vi "DAQ_Control.vi"(0 "Channel in":T3, 3 "Reading Cluster in":T1, 4 "Iteration Duration":i64) -> (5 "DAQ time":u32, 6 "Gradients":waveform(dbl)[](graph), 7 "cDAQ time":u32, 9 "Stop?":bool, 10 "Temps":waveform(dbl)[](graph), 11 "Time Left:":string, 12 "Camera Feed":T5, 13 "Output%":dbl(slide) caption="Cooling" scale=0.0..100.0 scale format="%.0f %", 14 "Channel out":T4, 15 "Readings out":T2, 17 "Reading Cluster":T1, 18 "DP_Overhead":i64(graph) caption="Data Acquisition - Overhead", 19 "Temp":dbl[unit] caption="Temperature" format="%.2f")   [LabVIEW 2024]
uses:
  <vilib>/vision/Image Controls.llb/IMAQ Image.ctl
  <extravilib>/ChannelInstances/Stream-str/)Channel.ctl
  <extravilib>/ChannelInstances/Tag-t'DataCluster.ctl'/))Channel.ctl
  DataCluster.ctl
  <vilib>/userDefined/High Color/IMAQdx.ctl
  <extravilib>/ChannelInstances/Tag-c(a[.](dbl),a[.](dbl))/))Channel.ctl
  <extravilib>/ChannelInstances/Tag-t'DataCluster.ctl'/Read With Abort.vi
  <extravilib>/ChannelInstances/Tag-c(a[.](dbl),a[.](dbl))/Write With Abort.vi
  <extravilib>/ChannelInstances/Tag-t'DataCluster.ctl'/EndpointRead.vi
  <extravilib>/ChannelInstances/Tag-c(a[.](dbl),a[.](dbl))/Endpoint.vi
  <extravilib>/ChannelInstances/Tag-t'DataCluster.ctl'.lvlib
  <extravilib>/ChannelInstances/Tag-c(a[.](dbl),a[.](dbl)).lvlib
  <extravilib>/ChannelInstances/Stream-str.lvlib
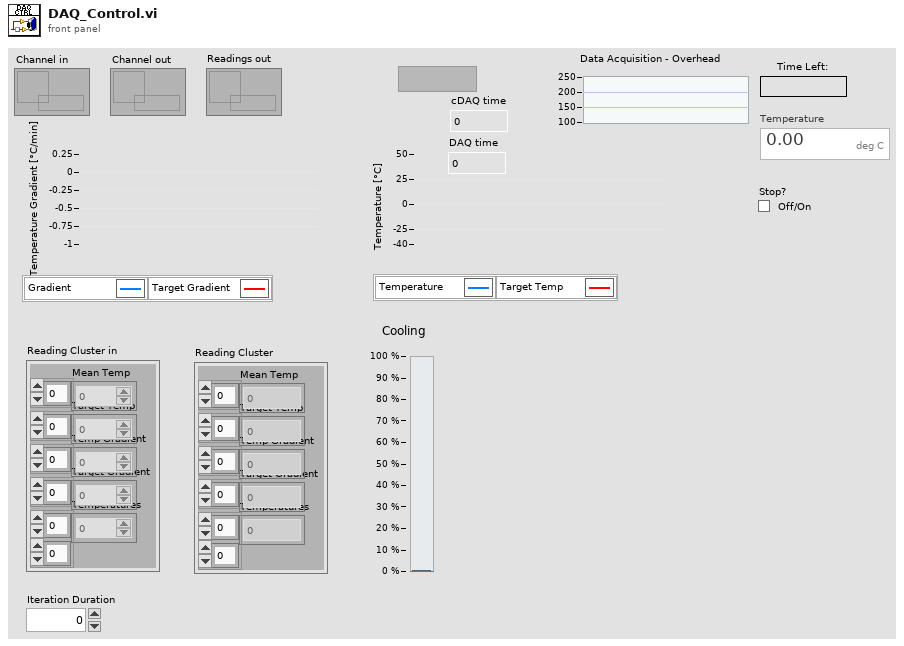
[diagram p1: front panel]
types:
  T1 = cluster{"Mean Temp":dbl[], "Target Temp":dbl[], "Temp Gradient":dbl[], "Target Gradient":dbl[], "Temperatures":dbl[][]}
  T2 = typedef "Tag-c(a[.](dbl),a[.](dbl)).lvlib/))Channel.ctl" = refnum<queue>
  T3 = typedef "Tag-t'DataCluster.ctl'.lvlib/))Channel.ctl" = refnum<queue>
  T4 = typedef "Stream-str.lvlib/)Channel.ctl" = refnum<queue>
  T5 = typedef "IMAQ Image.ctl" = refnum<image>
  T6 = typedef "DataCluster.ctl" = cluster{"Core":cluster{"Current VI Reference":refnum<vi>, "Close Panel on Exit?":bool, "Exit":bool, "Initialized?":bool}, "Connections":cluster{"cDAQ":cluster{"Task":refnum<k21>, "Connected":bool, "Active":bool, "ID":string}, "Camera":cluster{"Session":T7, "Connected":bool, "Active":bool, "Placeholder":T5}, "PSU":cluster{"Port":refnum<visa-resource-name>, "Connected":bool, "Active":bool}, "Arduino":cluster{"Port":refnum<visa-resource-name>, "Connected":bool, "Active":bool}}, "Data Acquisition":cluster{"Setup":cluster{"Label":string, "Operator":string, "Notes":string, "TempGrad":dbl, "TargetTemp":dbl, "Sample Volume":dbl}, "Camera":cluster{"Image":T5, "Save Image":T5, "Image Frequency":i32, "Rectangle":T8, "Calibration":cluster{"Top Left":T9, "Top Right":T9, "Bottom Left":T9, "Bottom Right":T9, "Fixpoint":T9, "Scan Area":dbl, "Fixpoint Area":dbl, "Well Pixels":cluster{"X":i32, "Y":i32}[][], "Valid":bool}, "FocusPos":u32, "Display Mapping":u32, "Camera Mode":u32}, "Thermistor":cluster{"Sample Size":i32, "Calibration":cluster{"B0.100":dbl[], "R25":dbl[], "c":dbl[][], "State":bool[], "V_S":dbl, "R_S":dbl}, "Timing Mode":i32}, "Partition":cluster{"Data":string[][], "Cell Label":string, "Cell Color":u32, "Height":i32, "Width":i32, "Grid":string[][]}, "Queue":cluster{"Size":i32, "Queue":refnum<queue>}, "Sample Rate":i32, "Active":bool, "Ready":bool, "Graph Mode":u16, "Gradient Buffer":i32}, "Control":cluster{"Sample Rate":i32, "PID gains":cluster{"proportional gain (Kc)":dbl, "integral time (Ti, min)":dbl, "derivative time (Td, min)":dbl}}, "Manual Temp Control":cluster{"TargetTemp":dbl, "Mode":u16, "Active":bool}}
  T7 = typedef "IMAQdx.ctl" = refnum<k21>
  T8 = typedef "IMAQ Rectangle" = cluster{"Left":i32, "Top":i32, "Right":i32, "Bottom":i32, "Rotation":dbl}
  T9 = typedef "IMAQ Point" = cluster{"X":sgl, "Y":sgl}
  T10 = cluster{"Temperature Readings Duplicate":dbl[], "Voltage Readings Duplicate":dbl[]}
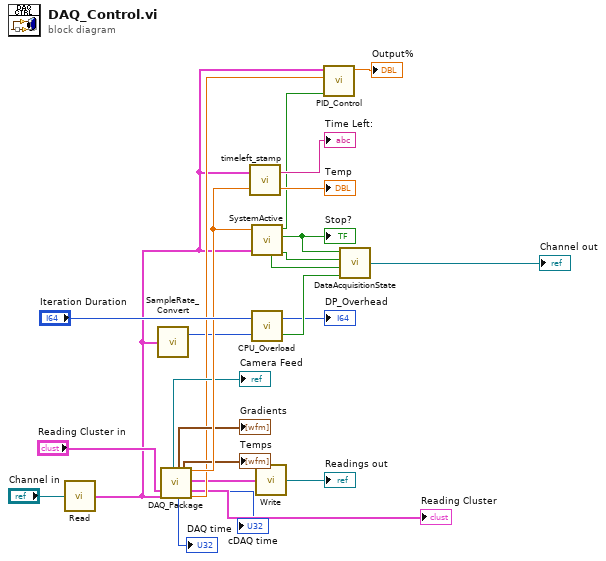
[diagram p0: block diagram]
diagram:
  n1 = call <extravilib>:"Read.vi"("channel"="Channel in") -> ("element"=w2:T6)  [unwired: 1 in, 1 out]
  n2 = call "SampleRate_Convert.vi"("DataCluster"=w2) -> ("Sample dt (ms)"=w10:i64)  [unwired: 1 out]
  n3 = call "DAQ_Package.vi"("Reading Cluster in"="Reading Cluster in", "Cluster in"=w2) -> ("Camera feed"=→"Camera Feed":T5, "Gradients Graph"=→"Gradients":waveform(dbl)[], "DAQ time"=→"DAQ time":u32, "Temps Graph"=→"Temps":waveform(dbl)[], "cDAQ time"=→"cDAQ time":u32, "Mean Temp Therm"=w18:dbl, "Readings out"=w9:T10, "Reading Cluster"=→"Reading Cluster":T1, "Temp Gradient"=w13:dbl)  [unwired: 9 in]
  n4 = call "timeleft_stamp.vi"("temp"=w18, "DataCluster"=w2) -> ("Temp"=→"Temp":dbl[unit], "time left"=→"Time Left:":string)
  n5 = call "SystemActive.vi"("DataCluster"=w2, "current temp"=w18) -> ("Temp reached"=w22:bool, "Above max Temp!"=w23:bool, "!Ready/!Active/Exit"=w6:bool, "reinit?"=w1:bool)  [unwired: 3 out]
  "Stop?" <- w6
  n6 = call "CPU_Overload.vi"("Sample dt"=w10, "Iteration Duration"="Iteration Duration") -> ("CPU_Overload?"=w24:bool, "DP_Overhead"=→"DP_Overhead":i64)
  n7 = call <extravilib>:"Write.vi"("element"=w9) -> ("channel"=→"Readings out":T2)  [unwired: 1 out]
  n8 = call "PID_Control.vi"("reinitialize? (F)"=w1, "Gradient"=w13, "DataCluster"=w2) -> ("Output%"=→"Output%":dbl)  [unwired: 8 in]
  n9 = call "DataAcquisitionState.vi"("CPU_Overload?"=w24, "Above max Temp!"=w23, "Temp reached"=w22, "Stop?"=w6) -> ("Channel out"=→"Channel out":T4)
